vi "Get URL.vi"(8 "Error In":errorcluster, 11 "object in":refnum<class "WebView.lvclass">) -> (0 "Error Out":errorcluster, 2 "URL":string, 3 "object out":refnum<class "WebView.lvclass">)   [LabVIEW 2024, in "WebView.lvclass"]
uses:
  <resource>/Framework/Providers/Open_GDS/ClassProviders/Provider_LvNativeClass/Templates/NativeBaseTemplate_4x4x4/NativeBaseTemplate_4x4x4.lvclass/NativeBaseTemplate_4x4x4.ctl
  WebView.lvclass
  WebView.lvclass/WebView.ctl
  <vilib>/sklein/WebView2/Libs/Microsoft.Web.WebView2.Core.dll
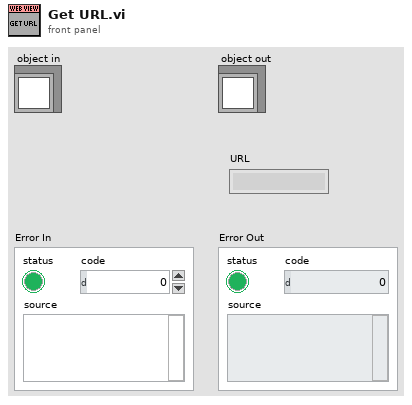
[diagram p1: front panel]
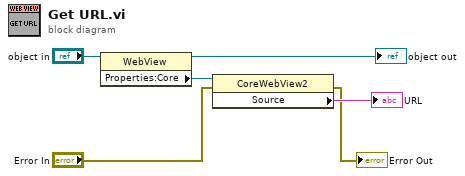
[diagram p0: block diagram]
diagram:
  n1 = property class="WebView"(reference="object in") -> (reference out=→"object out":refnum<class "WebView.lvclass">, "Properties:Core"=w4:refnum<k24>)  [unwired: 1 in, 1 out]
  n2 = property class="CoreWebView2"(reference=w4, error in="Error In") -> (error out=→"Error Out":errorcluster, "Source"=→"URL":string)  [unwired: 1 out]
